vi "get display name.vi"(8 "error in":errorcluster, 11 "cosmetic changes in":refnum<class "cosmetic changes.lvclass">) -> (0 "error out":errorcluster, 2 "class name":string, 3 "cosmetic changes out":refnum<class "cosmetic changes.lvclass">)   [LabVIEW 2013, in "cosmetic changes.lvclass"]
uses:
  cosmetic changes.lvclass
  VI modification.lvclass
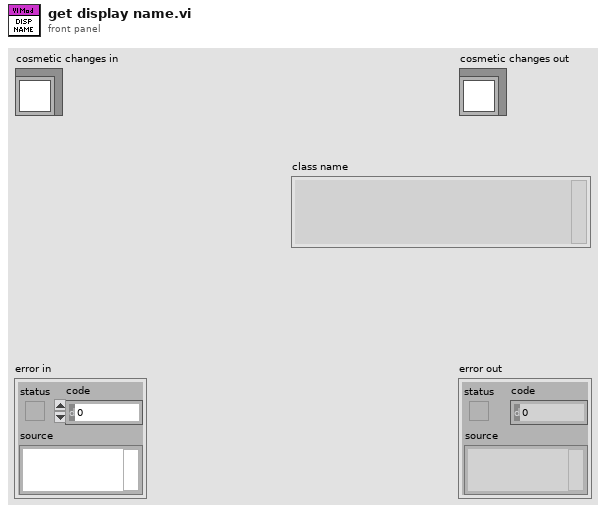
[diagram p1: front panel]
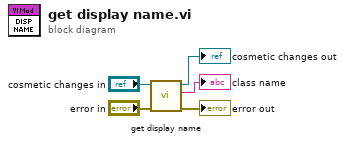
[diagram p0: block diagram]
diagram:
  n1 = call-parent "get display name.vi"("error in"="error in", "VI modification in"="cosmetic changes in") -> ("error out"=→"error out":errorcluster, "class name"=→"class name":string, "VI modification out"=→"cosmetic changes out":refnum<class "cosmetic changes.lvclass">)  [unwired: 7 in]
